vi "Read Buttons Def JSON.vi"(8 "error in":errorcluster, 10 "Button Def JSON":path) -> (0 "error out":errorcluster, 2 "Button Objects":T1[](array[typedef]))   [LabVIEW 2022 SP3, in "Navigation.lvlib" / "Button Manager.lvclass"]
doc: "____\nHAMPEL SOFTWARE ENGINEERING v2.6.0 (2023-12-19 10:54)"
uses:
  Button Manager.lvclass
  Top Control.ctl
  Sub Control.ctl
  Sidebar JSON Oject.ctl
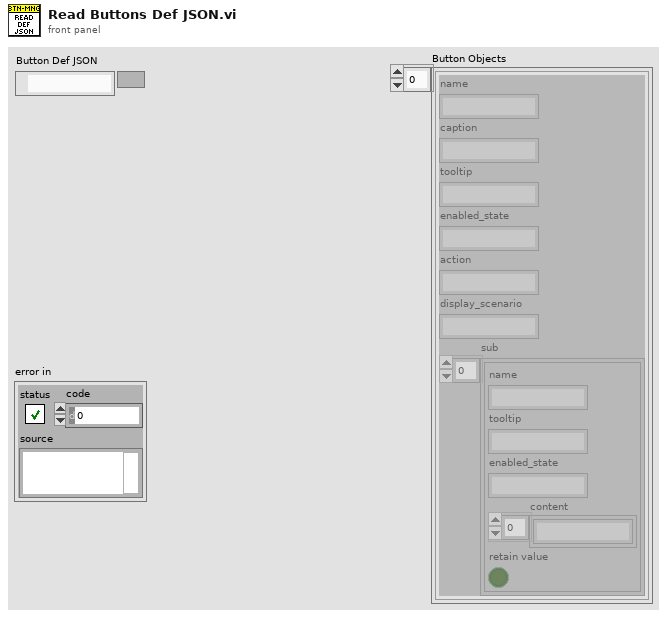
[diagram p1: front panel]
types:
  T1 = typedef "Navigation.lvlib/Button Manager.lvclass/Top Control.ctl" = cluster{"name":string, "caption":string, "tooltip":string, "enabled_state":string, "action":string, "display_scenario":string, "sub":T2[]}
  T2 = typedef "Navigation.lvlib/Button Manager.lvclass/Sub Control.ctl" = cluster{"name":string, "tooltip":string, "enabled_state":string, "content":string[], "retain value":bool}
  T3 = enum16{"open", "replace", "create", "open or create", "replace or create", "replace or create with confirmation"}
  T4 = typedef "Navigation.lvlib/Button Manager.lvclass/Sidebar JSON Oject.ctl" = cluster{"top":T1[]}
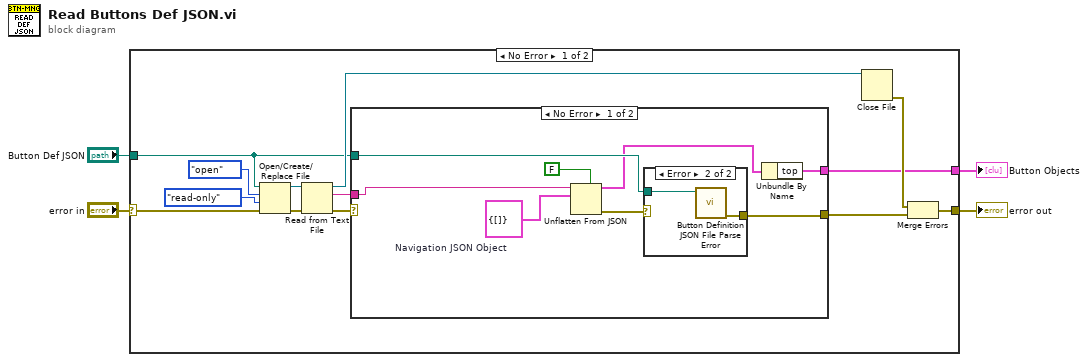
[diagram p0: block diagram]
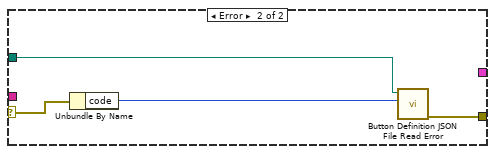
[diagram p3: hidden frame]
diagram:
  n1 = case shown="No Error" "error in" {
    selector: "error in" -> [w16 w32]
    tunnel: [w11 w32] -> w3
    tunnel: "Button Def JSON" -> [w5 _]
    tunnel: [w7 _] -> w1
    frame No Error {
      n2 = Open/Create/Replace File(file path (use dialog)=w5, error in=w16, operation (0:open)=T3."open", access (0:read/write)=enum16{"read/write", "read-only", "write-only"}."read-only") -> (refnum out=w12:refnum<file>, error out=w13:errorcluster)  [unwired: 2 in, 1 out]
      n3 = Read from Text File(file (use dialog)=w12, error in=w13) -> (refnum out=w6:refnum<file>, text=w8:string, error out=w10:errorcluster)  [unwired: 2 in, 1 out]
      n4 = case shown="No Error" w10 {
        selector: w10 -> [_ w31]
        tunnel: [w21 w28] -> w9
        tunnel: w8 -> [w25 _]
        tunnel: [w23 _] -> w7
        tunnel: w5 -> [w19 w29]
        frame No Error {
          w24 = T4 {"top"=[]}  # Navigation JSON Object
          n5 = Unflatten From JSON(enable LabVIEW extensions? (T)=FALSE, JSON string=w25, type and defaults=w24) -> (value=w18:T4, error out=w22:errorcluster)  [unwired: 4 in]
          n6 = case shown="Error" w22 {
            tunnel: [_ w27] -> w21
            tunnel: w19 -> [_ w26]
            frame No Error {
            }
            frame Error {
              n7 = call "Button Definition JSON File Parse Error.vi"("Button Def JSON"=w26) -> ("error out"=w27:errorcluster)  [unwired: 10 in]
            }
          }
          n8 = Unbundle By Name(w18) -> ("top"=w23:T1[])
        }
        frame Error {
          n9 = Unbundle By Name(w31) -> ("code"=w30:i32)
          n10 = call "Button Definition JSON File Read Error.vi"("error code"=w30, "Button Def JSON"=w29) -> ("error out"=w28:errorcluster)  [unwired: 9 in]
        }
      }
      n11 = Close File(refnum=w6) -> (error out=w17:errorcluster)  [unwired: 1 in, 1 out]
      n12 = Merge Errors(w17, w9) -> (w11:errorcluster)
    }
    frame Error {
    }
  }
  "error out" <- w3
  "Button Objects" <- w1
